vi "uTTA_ParseT3rFile.vi"(0 "uTTA_MeasureFile":string) -> (5 "Runtime ParseFile":dbl, 8 "uTTA_MeasureData":T1, 9 "uTTA_MetaData":T2 {"No Suspect Lines" format="%.3pV"; "Interpolation Factor m" format="%.2g"; "Interpolation Offset" format="%.2g"; "Chip Size" format="%.2gmm²"; "Heating Power" format="%.3pW"; "Cool Volt Deviation" format="%.3pV"; "Cool Voltage" format="%.3pV"})   [LabVIEW 2021]
uses:
  uTTA_MetaData.ctl
  CTL_uTTA_MeasurementDataValues.ctl
panel:
  out "SuspectLines":string[][](table)
  out "Samples/Decade":u32
  out "Tsamp,slow":dbl format="%#_g us"
  out "Tsamp,fast":dbl format="%#_g us"
  out "Total Blocks":u32
  out "Cooling Start Block":u32
  out "T_Cool":dbl format="%#_g s"
  out "T_Heat":dbl format="%#_g s"
  out "T_Preheat":dbl format="%#_g s"
  out "Max.Divider":u32
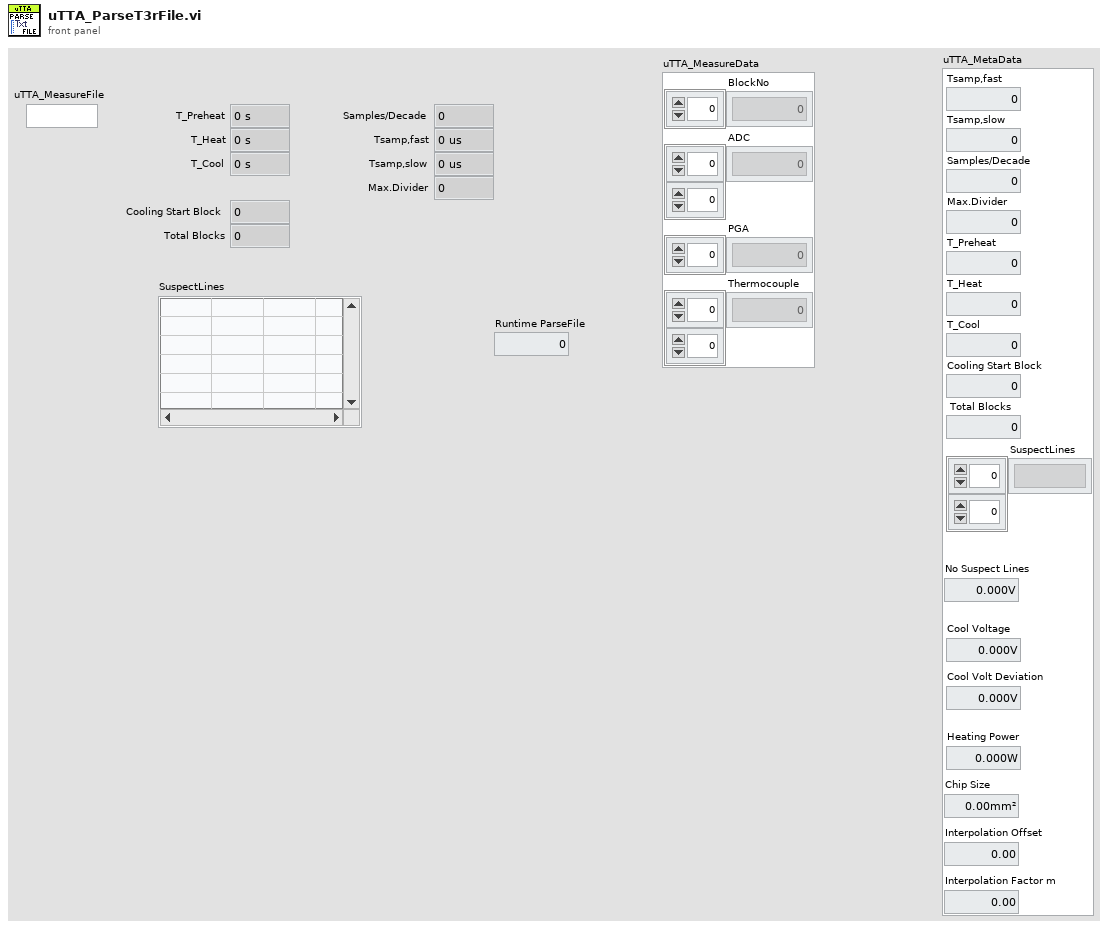
[diagram p1: front panel]
types:
  T1 = typedef "CTL_uTTA_MeasurementDataValues.ctl" = cluster{"BlockNo":i32[], "ADC":i32[][], "PGA":i32[], "Thermocouple":dbl[][]}
  T2 = typedef "uTTA_MetaData.ctl" = cluster{"Tsamp,fast":dbl, "Tsamp,slow":dbl, "Samples/Decade":u32, "Max.Divider":u32, "T_Preheat":dbl, "T_Heat":dbl, "T_Cool":dbl, "Cooling Start Block":u32, " Total Blocks":u32, "SuspectLines":string[][], "Cool Voltage":dbl, "Cool Volt Deviation":dbl, "Heating Power":dbl, "Chip Size":dbl, "Interpolation Offset":dbl, "Interpolation Factor m":dbl, "No Suspect Lines":u32}
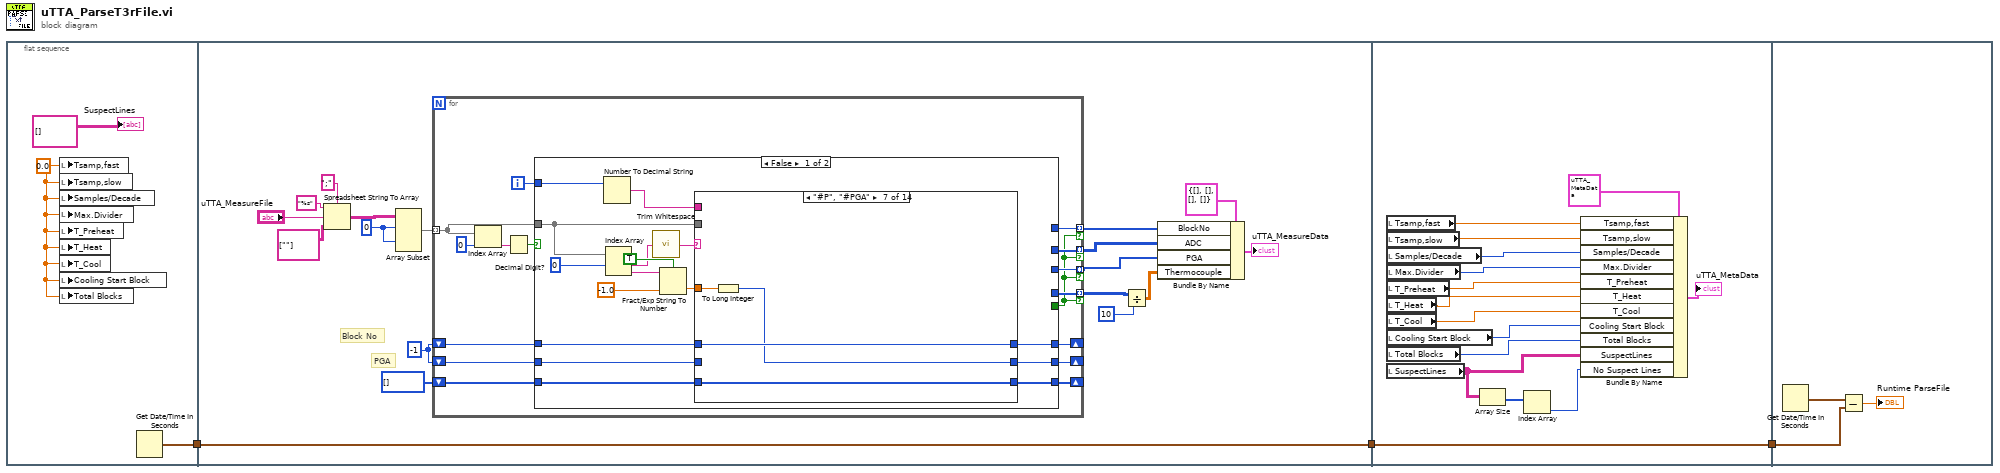
[diagram p0: block diagram]
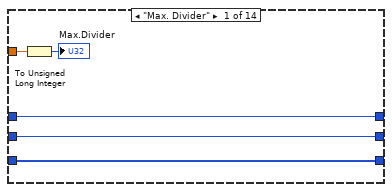
[diagram p2: hidden frame]
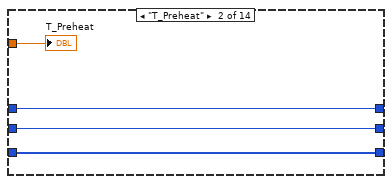
[diagram p3: hidden frame]
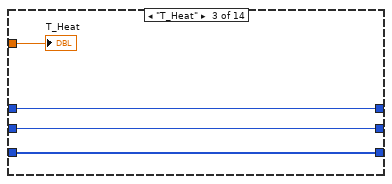
[diagram p4: hidden frame]
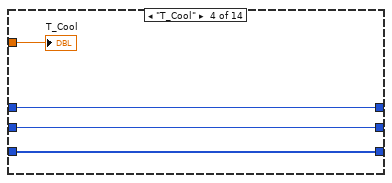
[diagram p5: hidden frame]
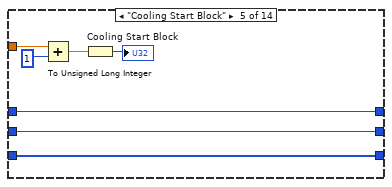
[diagram p6: hidden frame]
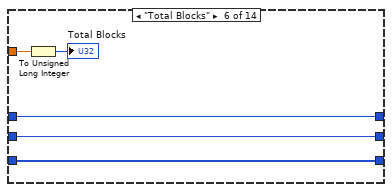
[diagram p7: hidden frame]
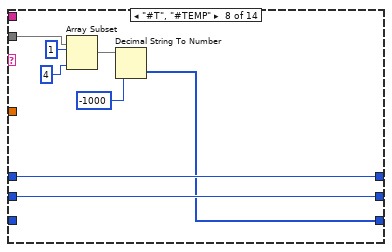
[diagram p8: hidden frame]
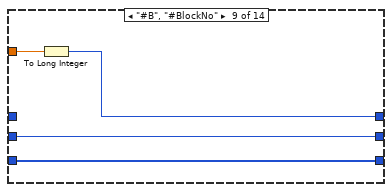
[diagram p9: hidden frame]
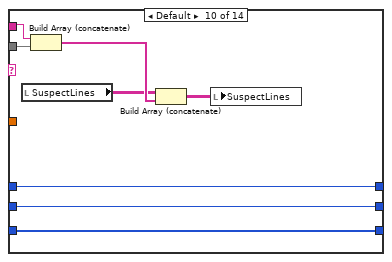
[diagram p10: hidden frame]
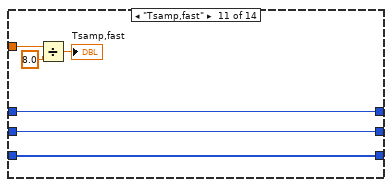
[diagram p11: hidden frame]
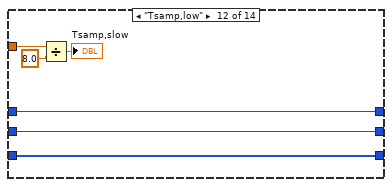
[diagram p12: hidden frame]
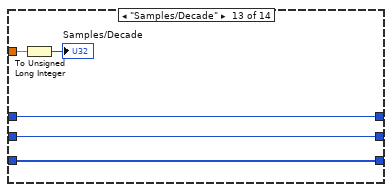
[diagram p13: hidden frame]
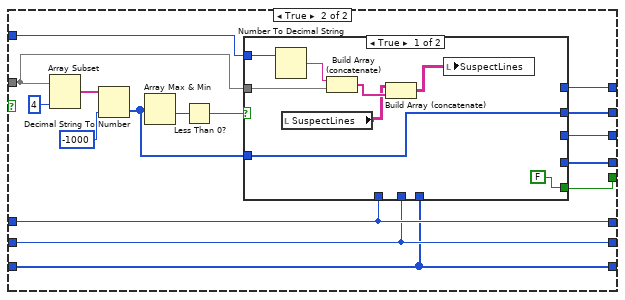
[diagram p15: hidden frame]
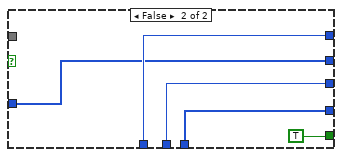
[diagram p16: hidden frame]
diagram:
  n1 = flat-sequence {
    tunnel: [w4] -> w3
    tunnel: w3 -> [w16]
    tunnel: [w16] -> w2
    tunnel: w2 -> [w164]
    tunnel: [w164] -> w1
    tunnel: w1 -> [w174]
    frame #0 {
      w5 = 0.0 ("Tsamp,fast")
      n2 = local write "Tsamp,fast"(w5) -> ()
      n3 = local write "Tsamp,slow"(w5) -> ()
      n4 = local write "Samples/Decade"(w5) -> ()
      n5 = local write "Max.Divider"(w5) -> ()
      n6 = local write "T_Preheat"(w5) -> ()
      n7 = local write "T_Heat"(w5) -> ()
      n8 = local write "T_Cool"(w5) -> ()
      n9 = local write "Cooling Start Block"(w5) -> ()
      n10 = local write "Total Blocks"(w5) -> ()
      n11 = Get Date/Time In Seconds() -> (seconds since 1Jan1904=w4:timestamp)
      "SuspectLines" <- string[][] [] ("SuspectLines")
    }
    frame #1 {
      w24 = -1 ("index")
      w21 = 0 ("index")
      # "PGA"
      # "Block No"
      n12 = Spreadsheet String To Array(delimiter (Tab)=";", format string="%s", spreadsheet string="uTTA_MeasureFile", array type (2D Dbl)=string[][] [[""]]) -> (array=w22:string[][])
      n13 = Array Subset(array=w22, index (row)=w21, index (col)=w21) -> (w23:string[][])  [unwired: 2 in]
      n14 = for {
        tunnel: w23 -> [w38] mode=indexing
        tunnel: [w40] -> w10 mode=indexing if=w25
        shift-right: [w32] -> _
        shift-left: w24 -> [w34]
        shift-right: [w31] -> _
        shift-left: w24 -> [w33]
        shift-right: [w30] -> _
        shift-left: i32[] [] -> [w29]
        tunnel: [w28] -> w11 mode=indexing if=w25
        tunnel: [w27] -> w9 mode=indexing if=w25
        tunnel: [w26] -> w13 mode=indexing if=w25
        i -> [w35]
        n15 = Index Array(array=w38, index=0) -> (element=w36:string)
        n16 = Decimal Digit?(1:w36) -> (0:w37:bool)
        n17 = case shown="False" w37 {
          tunnel: [_ w139] -> w40
          tunnel: w38 -> [w46 w134]
          tunnel: [_ w138] -> w25
          tunnel: w35 -> [w56 w142]
          tunnel: w34 -> [w54 w141]
          tunnel: w33 -> [w53 w140]
          tunnel: [w52 w141] -> w32
          tunnel: [w51 w140] -> w31
          tunnel: [w42 w133] -> w30
          tunnel: w29 -> [w41 w133]
          tunnel: [_ w132] -> w28
          tunnel: [_ w131] -> w27
          tunnel: [_ w130] -> w26
          frame False {
            n18 = Number To Decimal String(number=w56) -> (decimal integer string=w55:string)  [unwired: 1 in]
            n19 = Index Array(array=w46, index #1=0 ("index")) -> (element #1=w44:string, element #2=w43:string)  [unwired: 1 in]
            n20 = call <vilib>:"Trim Whitespace.vi"("string"=w44) -> ("trimmed string"=w47:string)  [unwired: 1 in]
            n21 = Fract/Exp String To Number(use system decimal point (T)=TRUE, string=w43, default (0 dbl)=-1.0 ("default (0 DBL)")) -> (number=w50:dbl)  [unwired: 1 in, 1 out]
            n22 = case shown="\"#P\", \"#PGA\"" w47 {
              tunnel: w50 -> [w61 w65 w69 w73 w80 w85 w88 _ w101 _ w114 w120 w126 _]
              tunnel: w46 -> [_ _ _ _ _ _ _ w92 _ w108 _ _ _ _]
              tunnel: w55 -> [_ _ _ _ _ _ _ _ _ w109 _ _ _ _]
              tunnel: w54 -> [w58 w63 w67 w71 w75 w82 w89 w97 _ w106 w111 w117 w123 w128]
              tunnel: w53 -> [w59 w64 w68 w72 w76 w83 _ w96 w99 w105 w112 w118 w124 w129]
              tunnel: [w58 w63 w67 w71 w75 w82 w89 w97 w100 w106 w111 w117 w123 w128] -> w52
              tunnel: [w59 w64 w68 w72 w76 w83 w87 w96 w99 w105 w112 w118 w124 w129] -> w51
              tunnel: [w57 w62 w66 w70 w74 w81 w86 w90 w98 w102 w110 w116 w122 w127] -> w42
              tunnel: w41 -> [w57 w62 w66 w70 w74 w81 w86 _ w98 w102 w110 w116 w122 w127]
              frame "Max. Divider" {
                n23 = To Unsigned Long Integer(number=w61) -> (unsigned 32bit integer=→"Max.Divider":u32)
              }
              frame "T_Preheat" {
                "T_Preheat" <- w65
              }
              frame "T_Heat" {
                "T_Heat" <- w69
              }
              frame "T_Cool" {
                "T_Cool" <- w73
              }
              frame "Cooling Start Block" {
                n24 = Add(x=w80, y=1) -> (x+y=w79:dbl)
                n25 = To Unsigned Long Integer(number=w79) -> (unsigned 32bit integer=→"Cooling Start Block":u32)
              }
              frame "Total Blocks" {
                n26 = To Unsigned Long Integer(number=w85) -> (unsigned 32bit integer=→"Total Blocks":u32)
              }
              frame "#P", "#PGA" {
                n27 = To Long Integer(number=w88) -> (32bit integer=w87:i32)
              }
              frame "#T", "#TEMP" {
                n28 = Array Subset(array=w92, index=1, length=4) -> (w95:string[])
                n29 = Decimal String To Number(string=w95, default (0L)=-1000 ("default (0 I32)")) -> (number=w90:i32[])  [unwired: 1 in, 1 out]
              }
              frame "#B", "#BlockNo" {
                n30 = To Long Integer(number=w101) -> (32bit integer=w100:i32)
              }
              frame Default {
                n31 = local read "SuspectLines"() -> (w103:string[][])
                n32 = Build Array (concatenate)(w109, w108) -> (w107:string[])
                n33 = Build Array (concatenate)(w103, w107) -> (w104:string[][])
                n34 = local write "SuspectLines"(w104) -> ()
              }
              frame "Tsamp,fast" {
                n35 = Divide(x=w114, y=8.0) -> (x/y=→"Tsamp,fast":dbl)
              }
              frame "Tsamp,low" {
                n36 = Divide(x=w120, y=8.0) -> (x/y=→"Tsamp,slow":dbl)
              }
              frame "Samples/Decade" {
                n37 = To Unsigned Long Integer(number=w126) -> (unsigned 32bit integer=→"Samples/Decade":u32)
              }
              frame "ADC1" {
              }
            }
          }
          frame True {
            n38 = Array Subset(array=w134, length=4) -> (w135:string[])  [unwired: 1 in]
            n39 = Decimal String To Number(string=w135, default (0L)=-1000 ("default (0 I32)")) -> (number=w137:i32[])  [unwired: 1 in, 1 out]
            n40 = Array Max & Min(array=w137) -> (min value=w144:i32)  [unwired: 3 out]
            n41 = Less Than 0?(x=w144) -> (x < 0?=w143:bool)
            n42 = case shown="True" w143 {
              tunnel: w134 -> [w153 _]
              tunnel: w142 -> [w151 _]
              tunnel: w141 -> [_ w157]
              tunnel: w140 -> [_ w155]
              tunnel: [w146 w156] -> w139
              tunnel: [FALSE TRUE] -> w138
              tunnel: w137 -> [w146 w156]
              tunnel: w133 -> [_ w154]
              tunnel: [_ w157] -> w132
              tunnel: [_ w155] -> w131
              tunnel: [_ w154] -> w130
              frame True {
                n43 = Number To Decimal String(number=w151) -> (decimal integer string=w150:string)  [unwired: 1 in]
                n44 = local read "SuspectLines"() -> (w147:string[][])
                n45 = Build Array (concatenate)(w150, w153) -> (w152:string[])
                n46 = Build Array (concatenate)(w147, w152) -> (w148:string[][])
                n47 = local write "SuspectLines"(w148) -> ()
              }
              frame False {
              }
            }
          }
        }
      }
      n48 = Divide(x=w13, y=10 ("index")) -> (x/y=w8:dbl[][])
      n49 = Bundle By Name(cluster=T1 {"BlockNo"=[], "ADC"=[], "PGA"=[], "Thermocouple"=[]}, "BlockNo"=w11, "ADC"=w10, "PGA"=w9, "Thermocouple"=w8) -> (→"uTTA_MeasureData":T1)
    }
    frame #2 {
      n50 = local read "Tsamp,fast"() -> (w173:dbl)
      n51 = local read "Tsamp,slow"() -> (w172:dbl)
      n52 = local read "Samples/Decade"() -> (w171:u32)
      n53 = local read "Max.Divider"() -> (w170:u32)
      n54 = local read "T_Preheat"() -> (w169:dbl)
      n55 = local read "T_Heat"() -> (w168:dbl)
      n56 = local read "T_Cool"() -> (w167:dbl)
      n57 = local read "Cooling Start Block"() -> (w166:u32)
      n58 = local read "Total Blocks"() -> (w165:u32)
      n59 = local read "SuspectLines"() -> (w161:string[][])
      n60 = Array Size(array=w161) -> (size(s)=w160:i32[])
      n61 = Index Array(array=w160) -> (element=w159:i32)  [unwired: 1 in]
      n62 = Bundle By Name(cluster=T2 {"Tsamp,fast"=1.25, "Tsamp,slow"=20480.0, "Samples/Decade"=200, "Max.Divider"=14, "T_Preheat"=60.0, "T_Heat"=2400.0, "T_Cool"=10800.0, "Cooling Start Block"=601, " Total Blocks"=3250, "SuspectLines"=[], "Cool Voltage"=0.0, "Cool Volt Deviation"=0.0, "Heating Power"=0.0, "Chip Size"=0.0, "Interpolation Offset"=0.0, "Interpolation Factor m"=0.0, "No Suspect Lines"=0} ("uTTA_MetaData"), "Tsamp,fast"=w173, "Tsamp,slow"=w172, "Samples/Decade"=w171, "Max.Divider"=w170, "T_Preheat"=w169, "T_Heat"=w168, "T_Cool"=w167, "Cooling Start Block"=w166, "Total Blocks"=w165, "SuspectLines"=w161, "No Suspect Lines"=w159) -> (→"uTTA_MetaData":T2)
    }
    frame #3 {
      n63 = Get Date/Time In Seconds() -> (seconds since 1Jan1904=w175:timestamp)
      n64 = Subtract(x=w175, y=w174) -> (x-y=→"Runtime ParseFile":dbl)
    }
  }
